vi "ReLU.vi"(1 "Z":T1) -> (0 "Relu":T1)   [LabVIEW 2016]
uses:
  <vilib>/Analysis/Matrix/Datatypes/RealMatrix.ctl
  <vilib>/Analysis/Matrix/Numeric/Conversions/Matrix To Array - RM.vi
  <vilib>/Analysis/Matrix/Numeric/Conversions/Array To Matrix - RA2.vi
  <vilib>/Analysis/Matrix/NI_Matrix.lvlib
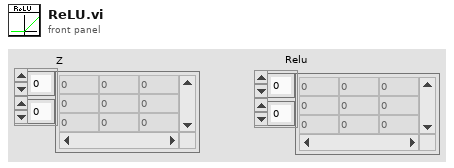
[diagram p1: front panel]
types:
  T1 = typedef "NI_Matrix.lvlib/RealMatrix.ctl" = dbl[][]
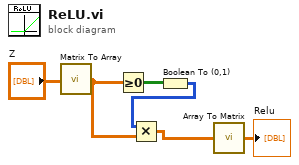
[diagram p0: block diagram]
diagram:
  n1 = call-poly <vilib>:"Matrix To Array.vi"("Real Matrix"="Z") -> ("Real 2D Array"=w3:dbl[][])
  n2 = Greater Or Equal To 0?(x=w3) -> (x >= 0?=w6:bool[][])
  n3 = Boolean To (0,1)(Boolean=w6) -> (0, 1=w5:i16[][])
  n4 = Multiply ("Multiply.vi")(x=w5, y=w3) -> (x*y=w2:dbl[][])
  n5 = call-poly <vilib>:"Array To Matrix.vi"("Real 2D Array"=w2) -> ("Real Matrix"=→"Relu":T1)
